vi "Send Pixel to FPGA.vi"(6 "Color":u16, 8 "error in":errorcluster, 9 "Y":u16, 10 "X":u16, 11 "FPGA VI Reference Out":T1) -> (0 "error out":errorcluster, 3 "FPGA VI Reference Out 2":T1)   [LabVIEW 2019]
uses:
  TypeDefs/FPGA Reference.ctl
  <vilib>/Utility/error.llb/Error Cluster From Error Code.vi
  <vilib>/rvi/errors/niLvFpgaAdjustHostInterfaceError.vi
  <vilib>/rvi/interface/nirviMethod/nirviMethod.xnode
  FPGA Bitfiles/adafruitlcdsom_FPGATarget_FPGAMain_K7l+4zj6vFY.lvbitx
  FPGA Main.vi
  <vilib>/FPGAPlugInAG/sbRIO-9651/niLvFpga_WriteFifo_sbRIO-9651.vi
  <vilib>/rvi/errors/niLvFpgaMergeErrorWithErrorCode.vi
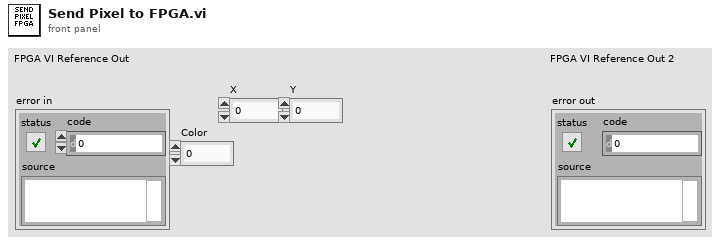
[diagram p1: front panel]
types:
  T1 = typedef "FPGA Reference.ctl" = refnum<k20>
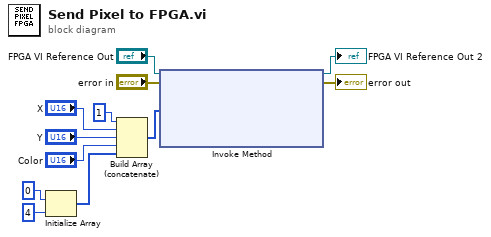
[diagram p0: block diagram]
diagram:
  n1 = Initialize Array(u16 0, 4 ("dimension size")) -> (w1:u16[])
  n2 = Build Array (concatenate)(u16 1 ("X"), "X", "Y", "Color", w1) -> (w3:u16[])
  n3 = xnode "Invoke Method"("FPGA VI Reference In"="FPGA VI Reference Out", "error in"="error in", "Data"=w3) -> ("FPGA VI Reference Out"=→"FPGA VI Reference Out 2":T1, "error out"=→"error out":errorcluster)  [unwired: 1 in, 1 out]
